vi "Keysight DAQ970-StatusSRQ.vi"() -> ()   [LabVIEW 2020, in "Keysight DAQ970.lvlib"]
doc: "This example program demonstrates how to setup the instrument status system to request service when a supported condition occurs and how to detect the SRQ using 2 techniques:\n1. Polling the instrument status byte \n2. Asynchronous SRQ event callback\n\nRuns in simulation mode without an instrument."
uses:
  Keysight DAQ970.lvlib
panel:
  in  "Write Buffer":u32[](array[numeric])=[42, 79, 80, 67]
  out "Output_Display":string
  out "Instrument":string[](array[string])
  out "Simulated":bool
  in  "Option String":string="DriverSetup= "
  in  "select":bool=TRUE
  in  "Resource String":string="MyVisaAlias"
  in  "Simulation":bool=TRUE caption="Simulate"
  # "Keysight DAQ970 - StatusSRQ"
  # "DRIVER REVISION"
  # "DRIVER VENDOR"
  # "DRIVER DESCRIPTION"
  # "INSTRUMENT MODEL"
  # "Simulate"
  # "Simulated"
  # "FIRMWARE REVISION"
  # "SERIAL NO"
  # "© Keysight Technologies 2020-2021"
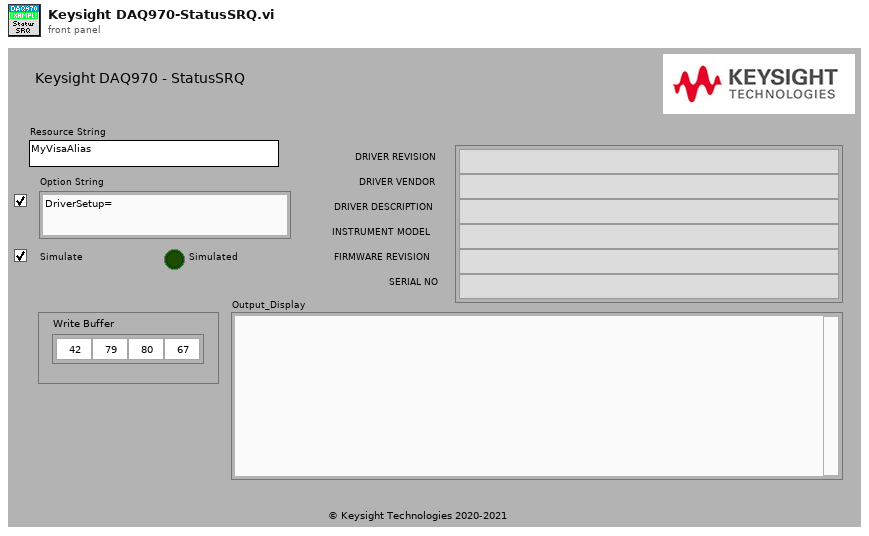
[diagram p1: front panel]
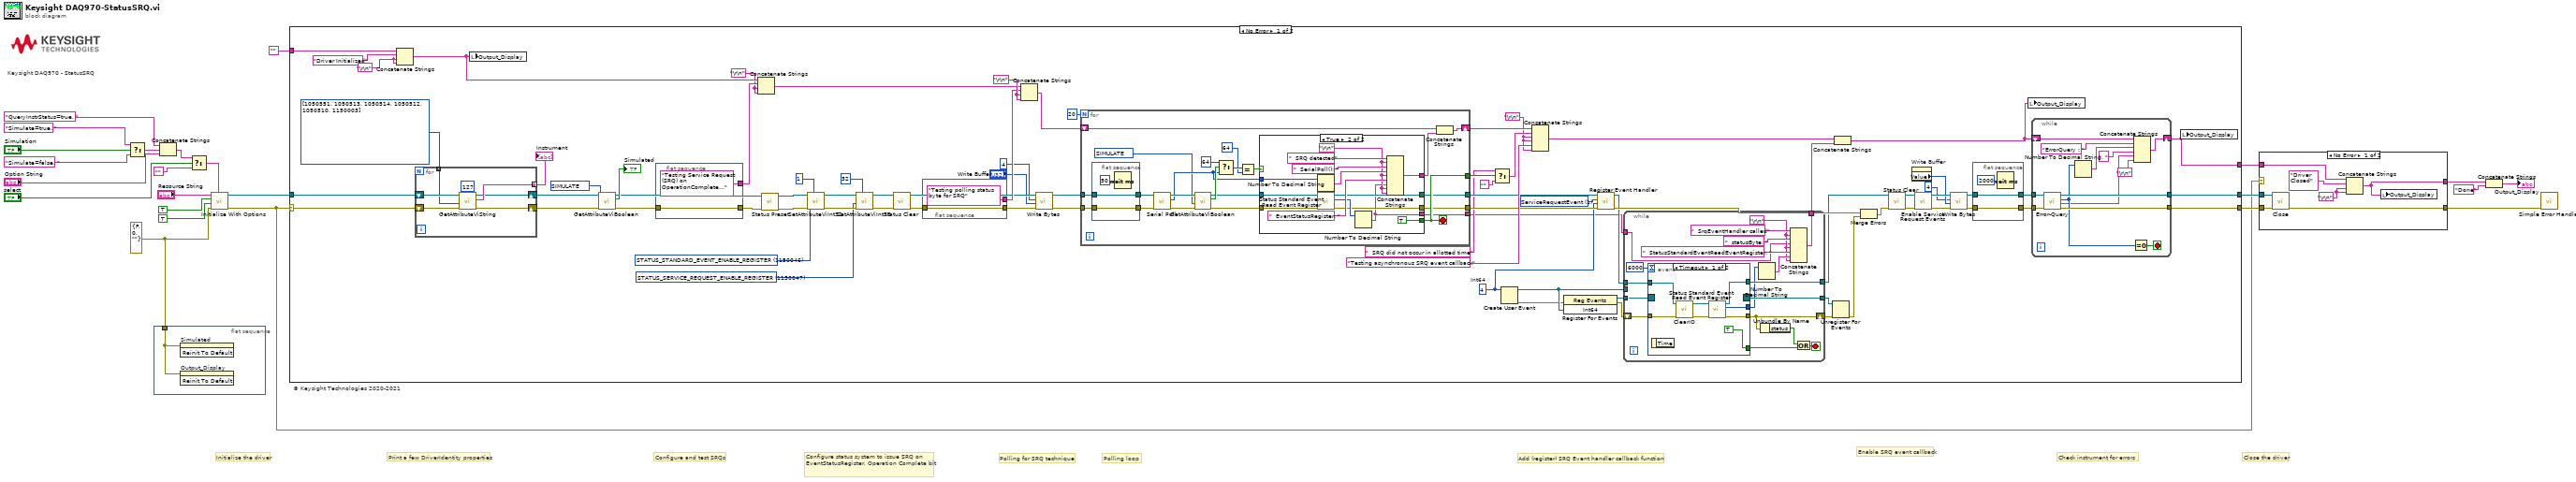
[diagram p0: block diagram]
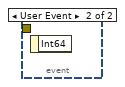
[diagram p3: hidden frame]
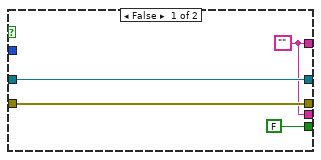
[diagram p4: hidden frame]
diagram:
  w3 = errorcluster {"status"=FALSE, "code"=0, "source"=""} ("error in (no error)")
  # "Enable SRQ event callback"
  # "Add (register) SRQ Event handler callback function"
  # "Configure and test SRQs"
  # "Polling for SRQ technique"
  # "Check instrument for errors"
  # "Configure status system to issue SRQ on EventStatusRegister, Operation Complete bit"
  # "Polling loop"
  # "Close the driver"
  # "Print a few DriverIdentity properties"
  # "© Keysight Technologies 2020-2021"
  # "Keysight DAQ970 - StatusSRQ"
  # "Initialize the driver"
  n1 = Select(t="Simulate=true, ", s="Simulation", f="Simulate=false, ") -> (s? t:f=w22:string)
  n2 = flat-sequence {
    tunnel: w3 -> [w25]
    frame #0 {
      n3 = invoke on="Simulated" class="Bool (strict)" method="Reinit To Default"(error in=w25) -> ()  [unwired: 2 in, 3 out]
      n4 = invoke on="Output_Display" class="Str" method="Reinit To Default"(error in=w25) -> ()  [unwired: 2 in, 3 out]
    }
  }
  n5 = Concatenate Strings("QueryInstrStatus=true, " ("string"), w22, "Option String") -> (w10:string)
  n6 = Select(t=w10, s="select", f="") -> (s? t:f=w7:string)
  n7 = call "Initialize With Options.vi"("option string"=w7, "error in (no error)"=w3, "reset device (Off)"=TRUE ("id query (Off)"), "id query (Off)"=TRUE, "resource string"="Resource String") -> ("error out"=w1:errorcluster, "instrument handle out"=w2:refnum<k15>)  [unwired: 5 in]
  n8 = case shown="No Error" w1 {
    selector: w1 -> [w98 w200]
    tunnel: w2 -> [w99 w202]
    tunnel: [w97 w202] -> w19
    tunnel: [w96 w200] -> w18
    tunnel: "" -> [w102 w201]
    tunnel: [w95 w201] -> w12
    frame No Error {
      w26 = u32 1050005 items=["DISPLAY_ENABLED"=1150016, "FORMAT_ALARM_ENABLED"=1150023, "FORMAT_CHANNEL_ENABLED"=1150024, "FORMAT_TIME_ENABLED"=1150025, "FORMAT_UNITS_ENABLED"=1150027, "ROUTE_MONITOR_ENABLED"=1150012, "SIMULATE"=1050005, "SYSTEM_AUTOCALIBRATION_GET_ALL_MODULE_STATE"=1150051, "SYSTEM_DMM_ENABLED"=1150018, "SYSTEM_DMM_INSTALLED"=1150019, "SYSTEM_INSTRUMENT_STATE_POWER_ON_RECALL_ENABLED"=1150033, "SYSTEM_LXI_IDENTIFY_ENABLED"=1150032, "SYSTEM_TRACING_ENABLED"=1150041, "USB_MEMORY_LOGGING_ENABLED"=1150034, "USB_MEMORY_MEASUREMENT_DATA_AUTO_SAVE_ENABLED"=1150057, "USB_MEMORY_RECALL_AUTO_ENABLED"=1150052, "USB_MEMORY_ROW_LIMIT_ENABLED"=1150036] ("AttributeID")
      w27 = u32 1150047 items=["ALARM_MODE"=1150006, "ALARM_SLOPE"=1150007, "FORMAT_TIME_MODE"=1150026, "ROUTE_MONITOR_VIEW"=1150068, "SCAN_CHANNEL_ADVANCE_SOURCE"=1150028, "SCAN_READING_THRESHOLD"=1150031, "SCAN_SINGLE_CHANNEL_SAMPLE_COUNT_PRE_TRIGGER"=1150063, "SCAN_SINGLE_CHANNEL_SAMPLE_COUNT"=1150062, "SCAN_SWEEP_COUNT"=1150008, "SCAN_TRIGGER_OUTPUT_SLOPE"=1150067, "SCAN_TRIGGER_SLOPE"=1150061, "SCAN_TRIGGER_SOURCE"=1150009, "STATUS_ALARM_ENABLE_REGISTER"=1150040, "STATUS_OPERATION_ENABLE_REGISTER"=1150044, "STATUS_QUESTIONABLE_ENABLE_REGISTER"=1150045, "STATUS_SERVICE_REQUEST_ENABLE_REGISTER"=1150047, "STATUS_STANDARD_EVENT_ENABLE_REGISTER"=1150046, "SYSTEM_AUTOCALIBRATION_MONTHLY_INTERVAL_DAY"=1150049, "SYSTEM_AUTOCALIBRATION_OCCURENCE_INTERVAL"=1150048, "SYSTEM_AUTOCALIBRATION_WEEKLY_INTERVAL_DAY"=1150050, "SYSTEM_IO_TIMEOUT"=1150002, "SYSTEM_TRACING_LEVEL"=1150043, "USB_MEMORY_COLUMN_HEADER"=1150054, "USB_MEMORY_COLUMN_SEPARATOR"=1150035, "USB_MEMORY_ROW_LIMIT_COUNT"=1150055] ("AttributeID")
      w28 = u32 1150046 items=["ALARM_MODE"=1150006, "ALARM_SLOPE"=1150007, "FORMAT_TIME_MODE"=1150026, "ROUTE_MONITOR_VIEW"=1150068, "SCAN_CHANNEL_ADVANCE_SOURCE"=1150028, "SCAN_READING_THRESHOLD"=1150031, "SCAN_SINGLE_CHANNEL_SAMPLE_COUNT_PRE_TRIGGER"=1150063, "SCAN_SINGLE_CHANNEL_SAMPLE_COUNT"=1150062, "SCAN_SWEEP_COUNT"=1150008, "SCAN_TRIGGER_OUTPUT_SLOPE"=1150067, "SCAN_TRIGGER_SLOPE"=1150061, "SCAN_TRIGGER_SOURCE"=1150009, "STATUS_ALARM_ENABLE_REGISTER"=1150040, "STATUS_OPERATION_ENABLE_REGISTER"=1150044, "STATUS_QUESTIONABLE_ENABLE_REGISTER"=1150045, "STATUS_SERVICE_REQUEST_ENABLE_REGISTER"=1150047, "STATUS_STANDARD_EVENT_ENABLE_REGISTER"=1150046, "SYSTEM_AUTOCALIBRATION_MONTHLY_INTERVAL_DAY"=1150049, "SYSTEM_AUTOCALIBRATION_OCCURENCE_INTERVAL"=1150048, "SYSTEM_AUTOCALIBRATION_WEEKLY_INTERVAL_DAY"=1150050, "SYSTEM_IO_TIMEOUT"=1150002, "SYSTEM_TRACING_LEVEL"=1150043, "USB_MEMORY_COLUMN_HEADER"=1150054, "USB_MEMORY_COLUMN_SEPARATOR"=1150035, "USB_MEMORY_ROW_LIMIT_COUNT"=1150055] ("AttributeID")
      w29 = u32[] [1050551, 1050513, 1050514, 1050512, 1050510, 1150003] items=["CALIBRATION_DATE"=1150065, "CALIBRATION_MESSAGE"=1150015, "CALIBRATION_TIME"=1150066, "DISPLAY_TEXT"=1150017, "DRIVER_SETUP"=1050007, "INSTRUMENT_FIRMWARE_REVISION"=1050510, "INSTRUMENT_MANUFACTURER"=1050511, "INSTRUMENT_MODEL"=1050512, "IO_RESOURCE_DESCRIPTOR"=1050304, "LOGICAL_NAME"=1050305, "ROUTE_MONITOR_CHANNEL"=1150010, "SCAN_LIST"=1150004, "SCAN_STARTTIME"=1150022, "SPECIFIC_DRIVER_DESCRIPTION"=1050514, "SPECIFIC_DRIVER_PREFIX"=1050302, "SPECIFIC_DRIVER_REVISION"=1050551, "SPECIFIC_DRIVER_VENDOR"=1050513, "SUPPORTED_INSTRUMENT_MODELS"=1050327, "SYSTEM_DATE"=1150020, "SYSTEM_SERIAL_NUMBER"=1150003, "SYSTEM_TIME"=1150021, "SYSTEM_TRACING_FILE_NAME"=1150042, "USB_MEMORY_DATA_FILE"=1150056, "USB_MEMORY_MEASUREMENTS_DATA_AUTO_SAVE_FILE"=1150058, "USB_MEMORY_SELECT_RECALL_AUTO_FILE"=1150053]
      w39 = i64 4  # Int64
      w62 = 1 items=["IviWarningEvent", "ServiceRequestEvent"] ("EventType (IviWarningEvent)")
      w51 = "\r\n"
      w76 = "\r\n"
      w88 = "\r\n"
      w100 = "\r\n"
      n9 = Concatenate Strings(w102, "Driver Initialized", w100, w100) -> (w90:string)
      n10 = for {
        tunnel: [w198] -> w103 mode=indexing
        shift-right: [w196] -> w94
        shift-left: w98 -> [w194]
        shift-right: [w197] -> w93
        shift-left: w99 -> [w195]
        tunnel: w29 -> [w193] mode=indexing
        n11 = call "GetAttributeViString.vi"("AttributeValueBufferSize"=127, "error in (no error)"=w194, "AttributeID"=w193, "instrument handle"=w195) -> ("error out"=w196:errorcluster, "AttributeValue"=w198:string, "instrument handle out"=w197:refnum<k15>)  [unwired: 5 in]
      }
      "Instrument" <- w103
      n12 = local write "Output_Display"(w90) -> ()
      n13 = call "GetAttributeViBoolean.vi"("error in (no error)"=w94, "AttributeID"=w26, "instrument handle"=w93) -> ("error out"=w91:errorcluster, "AttributeValue"=→"Simulated":bool, "instrument handle out"=w86:refnum<k15>)  [unwired: 6 in]
      n14 = flat-sequence {
        tunnel: w91 -> [w179]
        tunnel: [w179] -> w87
        tunnel: ["Testing Service Request (SRQ) on OperationComplete..."] -> w89
        frame #0 {
        }
      }
      n15 = Concatenate Strings(w90, w89, w88, w88) -> (w74:string)
      n16 = call "Status Preset.vi"("error in (no error)"=w87, "instrument handle"=w86) -> ("error out"=w85:errorcluster, "instrument handle out"=w84:refnum<k15>)  [unwired: 8 in]
      n17 = call "SetAttributeViInt32.vi"("AttributeValue"=1, "error in (no error)"=w85, "AttributeID"=w28, "instrument handle"=w84) -> ("error out"=w81:errorcluster, "instrument handle out"=w82:refnum<k15>)  [unwired: 6 in]
      n18 = call "SetAttributeViInt32.vi"("AttributeValue"=32, "error in (no error)"=w81, "AttributeID"=w27, "instrument handle"=w82) -> ("error out"=w79:errorcluster, "instrument handle out"=w78:refnum<k15>)  [unwired: 6 in]
      n19 = call "Status Clear.vi"("error in (no error)"=w79, "instrument handle"=w78) -> ("error out"=w77:errorcluster, "instrument handle out"=w72:refnum<k15>)  [unwired: 8 in]
      n20 = flat-sequence {
        tunnel: w77 -> [w176]
        tunnel: ["Testing polling status byte for SRQ"] -> w75
        tunnel: [w176] -> w73
        frame #0 {
        }
      }
      n21 = Concatenate Strings(w74, w75, w76, w76) -> (w67:string)
      n22 = call "Write Bytes.vi"("error in (no error)"=w73, "Buffer"="Write Buffer", "Count"=i64 4, "instrument handle"=w72) -> ("error out"=w68:errorcluster, "instrument handle out"=w69:refnum<k15>)  [unwired: 5 in, 1 out]
      n23 = for {
        N: 20 -> [_]
        tunnel: w69 -> [w151]
        tunnel: w68 -> [w150]
        shift-right: [w135] -> w66
        shift-left: w67 -> [w137]
        tunnel: [w134] -> w48
        tunnel: [w133] -> w50
        tunnel: [w132] -> w63
        tunnel: [w131] -> w33
        stop <- w134 stop-if-true
        w130 = u32 1050005 items=["DISPLAY_ENABLED"=1150016, "FORMAT_ALARM_ENABLED"=1150023, "FORMAT_CHANNEL_ENABLED"=1150024, "FORMAT_TIME_ENABLED"=1150025, "FORMAT_UNITS_ENABLED"=1150027, "ROUTE_MONITOR_ENABLED"=1150012, "SIMULATE"=1050005, "SYSTEM_AUTOCALIBRATION_GET_ALL_MODULE_STATE"=1150051, "SYSTEM_DMM_ENABLED"=1150018, "SYSTEM_DMM_INSTALLED"=1150019, "SYSTEM_INSTRUMENT_STATE_POWER_ON_RECALL_ENABLED"=1150033, "SYSTEM_LXI_IDENTIFY_ENABLED"=1150032, "SYSTEM_TRACING_ENABLED"=1150041, "USB_MEMORY_LOGGING_ENABLED"=1150034, "USB_MEMORY_MEASUREMENT_DATA_AUTO_SAVE_ENABLED"=1150057, "USB_MEMORY_RECALL_AUTO_ENABLED"=1150052, "USB_MEMORY_ROW_LIMIT_ENABLED"=1150036] ("AttributeID")
        n24 = flat-sequence {
          tunnel: [w171] -> w149
          tunnel: w151 -> [w171]
          tunnel: [w170] -> w148
          tunnel: w150 -> [w170]
          frame #0 {
            n25 = Wait (ms)(milliseconds to wait=u32 50) -> ()  [unwired: 1 out]
          }
        }
        n26 = call "Serial Poll.vi"("error in (no error)"=w148, "instrument handle"=w149) -> ("error out"=w146:errorcluster, "Val"=w140:i32, "instrument handle out"=w147:refnum<k15>)  [unwired: 7 in]
        n27 = call "GetAttributeViBoolean.vi"("error in (no error)"=w146, "AttributeID"=w130, "instrument handle"=w147) -> ("error out"=w138:errorcluster, "AttributeValue"=w145:bool, "instrument handle out"=w139:refnum<k15>)  [unwired: 6 in]
        n28 = Select(t=64, s=w145, f=w140) -> (s? t:f=w143:i32)
        n29 = Equal?(x=w143, y=64 ("value")) -> (x = y?=w141:bool)
        n30 = case shown="True" w141 {
          tunnel: w140 -> [_ w169]
          tunnel: w139 -> [w154 w165]
          tunnel: w138 -> [w153 w164]
          tunnel: [w152 w160] -> w136
          tunnel: [FALSE TRUE] -> w134
          tunnel: [w154 w158] -> w133
          tunnel: [w153 w157] -> w132
          tunnel: [w152 w156] -> w131
          frame False {
            w152 = ""
          }
          frame True {
            w161 = "\r\n"
            n31 = Number To Decimal String(number=w169) -> (decimal integer string=w166:string)  [unwired: 1 in]
            n32 = call "Status Standard Event Read Event Register.vi"("error in (no error)"=w164, "instrument handle"=w165) -> ("error out"=w157:errorcluster, "Val"=w162:i32, "instrument handle out"=w158:refnum<k15>)  [unwired: 7 in]
            n33 = Number To Decimal String(number=w162) -> (decimal integer string=w156:string)  [unwired: 1 in]
            n34 = Concatenate Strings("  SRQ detected" ("string"), w161, "  SerialPoll(): " ("string"), w166, w161, "  EventStatusRegister: " ("string"), w156, w161, w161) -> (w160:string)
          }
        }
        n35 = Concatenate Strings(w137, w136) -> (w135:string)
      }
      n36 = Select(t="  SRQ did not occur in allotted time" ("string"), s=w48, f="") -> (s? t:f=w65:string)
      n37 = Create User Event(user event datatype=w39) -> (user event=w44:refnum<user-event>, error out=w40:errorcluster)  [unwired: 1 in]
      n38 = Concatenate Strings(w66, w65, w51, w51, "Testing asynchronous SRQ event callback" ("string"), w51) -> (w31:string)
      n39 = register-events(error in=w40, w44) -> (reference out=w43:refnum<event-registration>, error out=w41:errorcluster)  [unwired: 1 in]
      n40 = call "Register Event Handler.vi"("error in (no error)"=w63, "CallbackFunctionPointer"=w39, "EventType (IviWarningEvent)"=w62, "instrument handle"=w50) -> ("error out"=w38:errorcluster, "instrument handle out"=w35:refnum<k15>)  [unwired: 6 in]
      n41 = while {
        tunnel: w43 -> [w121]
        shift-right: [w119] -> w45
        shift-left: w41 -> [w120]
        tunnel: w44 -> [_]
        tunnel: [w116] -> w42
        tunnel: w35 -> [w113]
        tunnel: [w112] -> w34
        tunnel: w33 -> [w105]
        tunnel: [w104] -> w32
        stop <- w117 stop-if-true
        w106 = "\r\n"
        n42 = event shown="[0] Timeout" {
          selector: w121 -> [_ _]
          dyn-events: [_ _] -> w116
          timeout: 6000 -> [_ _]
          tunnel: [TRUE ("Time has Elapsed") _] -> w118
          tunnel: w120 -> [w126 _]
          tunnel: [w125 _] -> w119
          tunnel: w113 -> [w124 _]
          tunnel: [w123 _] -> w112
          tunnel: [w122 _] -> w108
          event Timeout {
            n43 = event-data() -> ()  [unwired: 1 in, 1 out]
            n44 = call "ClearIO.vi"("error in (no error)"=w126, "instrument handle"=w124) -> ("error out"=w127:errorcluster, "instrument handle out"=w128:refnum<k15>)  [unwired: 8 in]
            n45 = call "Status Standard Event Read Event Register.vi"("error in (no error)"=w127, "instrument handle"=w128) -> ("error out"=w125:errorcluster, "Val"=w122:i32, "instrument handle out"=w123:refnum<k15>)  [unwired: 7 in]
          }
          event User Event {
            n46 = event-data() -> ()  [unwired: 1 in, 1 out]
          }
        }
        n47 = Number To Decimal String(number=w108) -> (decimal integer string=w107:string)  [unwired: 1 in]
        n48 = Unbundle By Name(w119) -> ("status"=w115:bool)
        n49 = Concatenate Strings("  SrqEventHandler called" ("string"), w106, "  statusByte: " ("string"), w105, w106, "  StatusStandardEventReadEventRegister: " ("string"), w107, w106) -> (w104:string)
        n50 = Or(x=w115, y=w118) -> (x .or. y?=w117:bool)
      }
      n51 = Unregister For Events(event registration refnum=w42, error in=w45) -> (error out=w37:errorcluster)
      n52 = Concatenate Strings(w31, w32) -> (w30:string)
      n53 = Merge Errors(w38, w37) -> (w36:errorcluster)
      n54 = call "Status Clear.vi"("error in (no error)"=w36, "instrument handle"=w34) -> ("error out"=w61:errorcluster, "instrument handle out"=w60:refnum<k15>)  [unwired: 8 in]
      n55 = property on="Write Buffer" class="Arr (strict)"() -> ("Value"=w57:u32[])  [unwired: 2 in, 2 out]
      n56 = call "Enable Service Request Events.vi"("error in (no error)"=w61, "instrument handle"=w60) -> ("error out"=w59:errorcluster, "instrument handle out"=w58:refnum<k15>)  [unwired: 8 in]
      n57 = call "Write Bytes.vi"("error in (no error)"=w59, "Buffer"=w57, "Count"=i64 4, "instrument handle"=w58) -> ("error out"=w54:errorcluster, "instrument handle out"=w55:refnum<k15>)  [unwired: 5 in, 1 out]
      n58 = flat-sequence {
        tunnel: [w174] -> w53
        tunnel: w55 -> [w174]
        tunnel: [w173] -> w52
        tunnel: w54 -> [w173]
        frame #0 {
          n59 = Wait (ms)(milliseconds to wait=u32 2000) -> ()  [unwired: 1 out]
        }
      }
      n60 = local write "Output_Display"(w30) -> ()
      n61 = while {
        tunnel: [w192] -> w96
        tunnel: [w191] -> w97
        shift-right: [w184] -> w95
        shift-left: w30 -> [w182]
        tunnel: w53 -> [w181]
        tunnel: w52 -> [w180]
        stop <- w190 stop-if-true
        n62 = call "Error-Query.vi"("error in (no error)"=w180, "instrument handle"=w181) -> ("error out"=w192:errorcluster, "error message"=w185:string, "error code"=w188:i32, "instrument handle out"=w191:refnum<k15>)  [unwired: 6 in]
        n63 = Number To Decimal String(number=w188) -> (decimal integer string=w187:string)  [unwired: 1 in]
        n64 = Equal To 0?(x=w188) -> (x = 0?=w190:bool)
        n65 = Concatenate Strings(w182, "ErrorQuery : ", w187, ", ", w185, "\r\n") -> (w184:string)
      }
      n66 = local write "Output_Display"(w95) -> ()
    }
    frame Error {
    }
  }
  n67 = case shown="No Error" w1 {
    tunnel: w19 -> [w204 _]
    tunnel: w18 -> [w205 w211]
    tunnel: [w208 w210] -> w16
    tunnel: [w203 w211] -> w13
    tunnel: w12 -> [w207 w210]
    frame No Error {
      w206 = "\r\n"
      n68 = call "Close.vi"("error in (no error)"=w205, "instrument handle"=w204) -> ("error out"=w203:errorcluster)  [unwired: 9 in]
      n69 = Concatenate Strings(w207, "Driver Closed", w206, w206) -> (w208:string)
      n70 = local write "Output_Display"(w208) -> ()
    }
    frame Error {
    }
  }
  n71 = Concatenate Strings(w16, "Done") -> (→"Output_Display":string)
  n72 = call <vilib>:"Simple Error Handler.vi"("error in (no error)"=w13) -> ()  [unwired: 4 in, 5 out]
